vi "MatchEmbedByGUID.vi"(8 "error in (no error)":errorcluster, 10 "GUID":string, 11 "SMO.UI.MAUI in":refnum<class "SMO.UI.MAUI.lvclass">) -> (0 "error out":errorcluster, 1 "Index":i32, 2 "Value":refnum<class "SMO.UI.Embedded.lvclass">, 3 "SMO.UI.MAUI out":refnum<class "SMO.UI.MAUI.lvclass">, 4 "Found?":bool)   [LabVIEW 2020, in "SMO.UI.MAUI.lvclass"]
uses:
  SMO.UI.MAUI.lvclass
  <vilib>/Levylab/SMO.UI.Embedded/SMO.UI.Embedded.lvclass
  C:/Program Files (x86)/National Instruments/LabVIEW 2020/vi.lib/JKI/JKI SMO/SMO/SMO.lvclass
  SMO.UI.MAUI.lvclass/SMO.UI.MAUI.ctl
  <vilib>/JKI/JKI SMO/SMO/SMO.lvclass
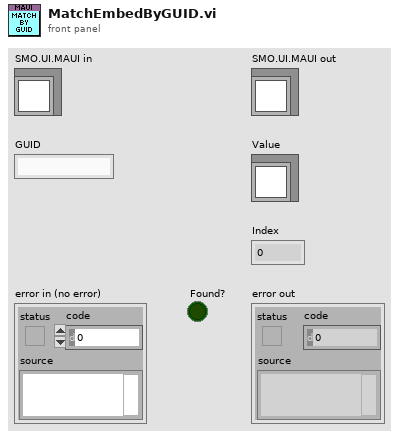
[diagram p1: front panel]
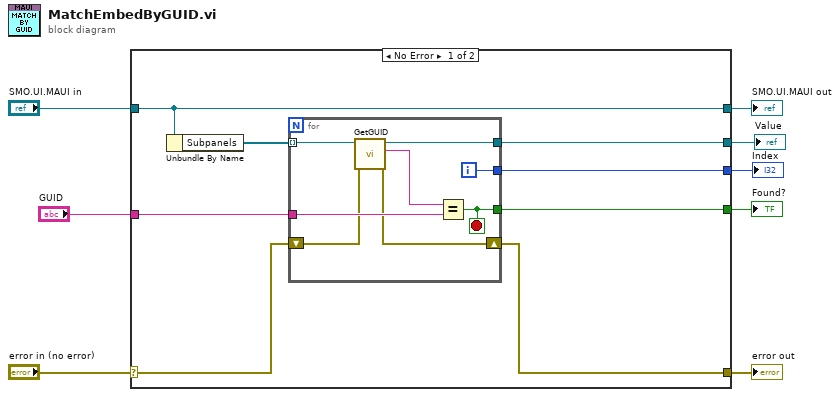
[diagram p0: block diagram]
diagram:
  n1 = case shown="No Error" "error in (no error)" {
    selector: "error in (no error)" -> [w13 w26]
    tunnel: [w12 w26] -> w7
    tunnel: [w16 w25] -> w5
    tunnel: "SMO.UI.MAUI in" -> [w16 w25]
    tunnel: "GUID" -> [w14 _]
    tunnel: [w11 _] -> w3
    tunnel: [w10 _] -> w2
    tunnel: [w9 _] -> w1
    frame No Error {
      n2 = Unbundle By Name(w16) -> ("Subpanels"=w15:refnum<class "SMO.UI.Embedded.lvclass">[])
      n3 = for {
        tunnel: w15 -> [w24] mode=indexing
        tunnel: w14 -> [w22]
        shift-right: [w20] -> w12
        shift-left: w13 -> [w21]
        tunnel: [w19] -> w10
        tunnel: [w18] -> w11
        tunnel: [w17] -> w9
        i -> [w19]
        stop <- w17 stop-if-true
        n4 = call <vilib>:"GetGUID.vi"("error in (no error)"=w21, "SMO"=w24) -> ("error out"=w20:errorcluster, "GUID"=w23:string, "SMO out"=w18:refnum<class "SMO.UI.Embedded.lvclass">)  [unwired: 7 in]
        n5 = Equal?(x=w23, y=w22) -> (x = y?=w17:bool)
      }
    }
    frame Error {
    }
  }
  "error out" <- w7
  "SMO.UI.MAUI out" <- w5
  "Value" <- w3
  "Index" <- w2
  "Found?" <- w1
